vi "FindVIAndReadControlValue.vi"(5 "Read Control Name":string, 7 "Running":bool=TRUE, 8 "Compare JSON value":string, 9 "Compare Control Name":string, 11 "VI Name regexp":string) -> (2 "Found":bool, 3 "Read Control Value":variant)   [LabVIEW 2021]
uses:
  <vilib>/regexp/Match Regular Expression.xnode
  SetGetControlValue.lvlib
panel:
  # "指定の条件を満たす VI を発見して\nコントロールの値を返す"
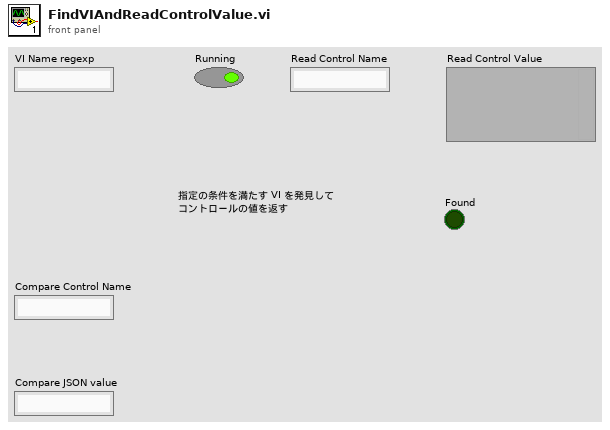
[diagram p1: front panel]
types:
  T1 = enum32{"Bad", "Idle", "Run top level", "Running"}
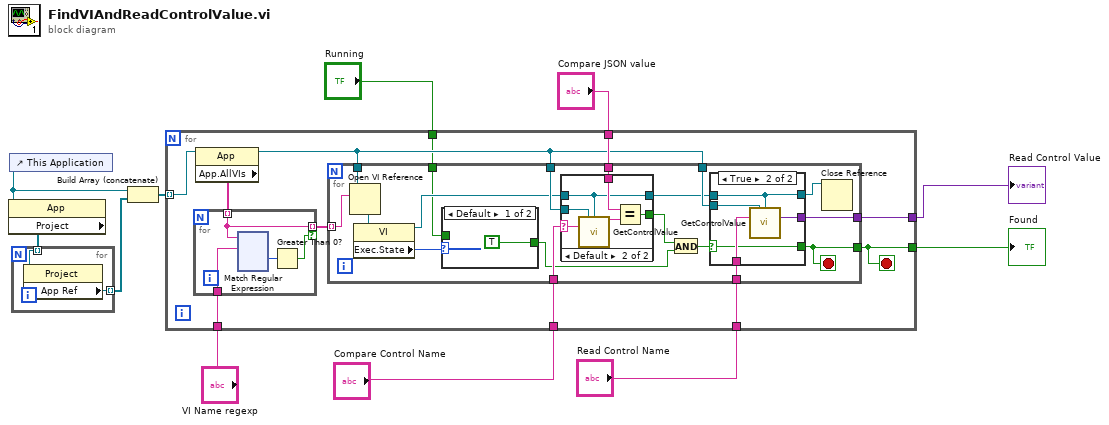
[diagram p0: block diagram]
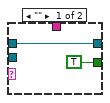
[diagram p2: hidden frame]
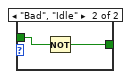
[diagram p3: hidden frame]
diagram:
  n1 = control-ref of="This Application"() -> (w3:refnum<vi>)
  n2 = property class="App"(reference=w3) -> ("Project"=w4:refnum<vi>[])  [unwired: 1 in, 2 out]
  n3 = for {
    tunnel: w4 -> [w13] mode=indexing
    tunnel: [w12] -> w5 mode=indexing
    n4 = property class="Project"(reference=w13) -> ("App Ref"=w12:refnum<vi>)  [unwired: 1 in, 2 out]
  }
  n5 = Build Array (concatenate)(w3, w5) -> (w6:refnum<vi>[])
  n6 = for {
    tunnel: w6 -> [w22] mode=indexing
    tunnel: "VI Name regexp" -> [w21]
    tunnel: "Compare Control Name" -> [w20]
    tunnel: "Compare JSON value" -> [w19]
    tunnel: [w18] -> w9
    tunnel: "Read Control Name" -> [w17]
    tunnel: [w16] -> w2
    tunnel: "Running" -> [w14]
    stop <- w16 stop-if-true
    n7 = property class="App"(reference=w22) -> (reference out=w15:refnum<vi>, "App.AllVIs"=w24:string[])  [unwired: 1 in, 1 out]
    n8 = for {
      tunnel: w24 -> [w62] mode=indexing
      tunnel: [w62] -> w23 mode=indexing if=w61
      tunnel: w21 -> [w60]
      n9 = xnode "Match Regular Expression"("input string"=w62, "regular expression"=w60) -> ("offset past match"=w63:i32)  [unwired: 4 in, 4 out]
      n10 = Greater Than 0?(x=w63) -> (x > 0?=w61:bool)
    }
    n11 = for {
      tunnel: w23 -> [w35] mode=indexing
      tunnel: w15 -> [w40]
      tunnel: w20 -> [w27]
      tunnel: w19 -> [w41]
      tunnel: [w39] -> w18
      tunnel: [w38] -> w16
      tunnel: w17 -> [w37]
      tunnel: w15 -> [w36]
      tunnel: w15 -> [w31]
      tunnel: w14 -> [w29]
      stop <- w38 stop-if-true
      n12 = Open VI Reference(application reference (local)=w36, vi path=w35) -> (vi reference=w34:refnum<vi>)  [unwired: 4 in, 1 out]
      n13 = property class="VI"(reference=w34) -> (reference out=w32:refnum<vi>, "Exec.State"=w30:T1)  [unwired: 1 in, 1 out]
      n14 = case shown="Default" w30 {
        tunnel: [TRUE w52] -> w26
        tunnel: w29 -> [_ w53]
        frame Default {
        }
        frame "Bad", "Idle" {
          n15 = Not(x=w53) -> (.not. x?=w52:bool)
        }
      }
      n16 = case shown="Default" w27 {
        selector: w27 -> [_ w46]
        tunnel: [TRUE w50] -> w42
        tunnel: w41 -> [_ w49]
        tunnel: w40 -> [_ w47]
        tunnel: w32 -> [w43 w45]
        tunnel: [w43 w45] -> w25
        frame "" {
        }
        frame Default {
          n17 = call "GetControlValue.vi"("application reference (local)"=w47, "vi ref"=w45, "ctrl"=w46) -> ("String out"=w48:string)  [unwired: 10 in, 2 out]
          n18 = Equal?(x=w49, y=w48) -> (x = y?=w50:bool)
        }
      }
      n19 = And(x=w42, y=w26) -> (x .and. y?=w28:bool)
      n20 = case shown="True" w28 {
        selector: w28 -> [_ w56]
        tunnel: w37 -> [_ w59]
        tunnel: w31 -> [_ w58]
        tunnel: [_ w57] -> w39
        tunnel: [_ w56] -> w38
        tunnel: w25 -> [w54 w55]
        tunnel: [w54 w55] -> w33
        frame False {
        }
        frame True {
          n21 = call "GetControlValue.vi"("application reference (local)"=w58, "vi ref"=w55, "ctrl"=w59) -> ("value"=w57:variant)  [unwired: 10 in, 2 out]
        }
      }
      n22 = Close Reference(reference=w33) -> ()  [unwired: 1 in, 1 out]
    }
  }
  "Read Control Value" <- w9
  "Found" <- w2
